vi "log_data_calibration.vi"(0 "Calibration":T1, 3 "error in (no error)":errorcluster, 4 "Elements Remaining":u32, 5 "Data":fxp<+/-,24,4>[](array[numeric])) -> (7 "number of elements out":u32, 10 "error out":errorcluster)   [LabVIEW 2015]
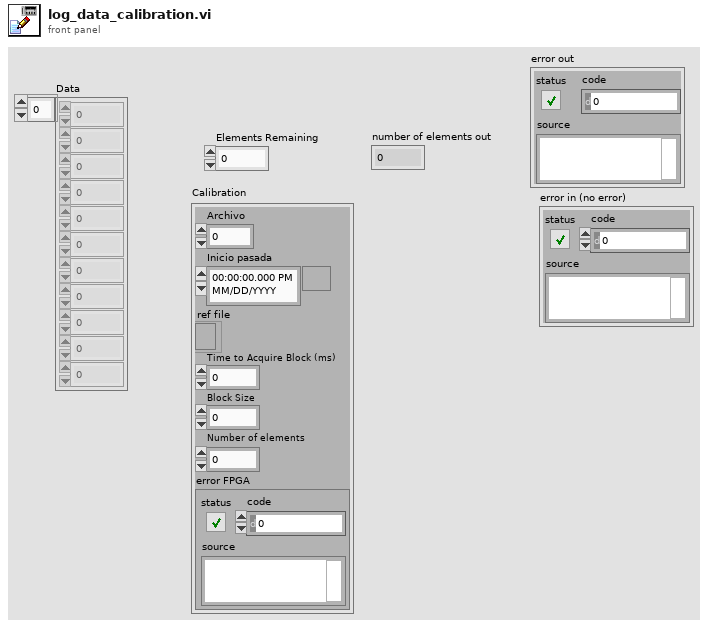
[diagram p1: front panel]
types:
  T1 = cluster{"Archivo":dbl, "Inicio pasada ":timestamp, "ref file":refnum<file>, "Time to Acquire Block (ms)":i32, "Block Size":u32, "Number of elements":u32, "error FPGA":errorcluster}
  T2 = enum16{"big-endian, network order", "native, host order", "little-endian"}
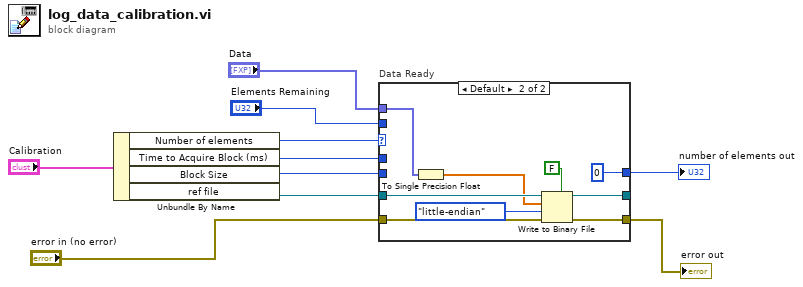
[diagram p0: block diagram]
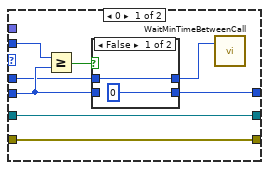
[diagram p2: hidden frame]
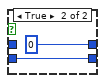
[diagram p3: hidden frame]
diagram:
  n1 = Unbundle By Name("Calibration") -> ("Number of elements"=w6:u32, "Time to Acquire Block (ms)"=w5:i32, "Block Size"=w4:u32, "ref file"=w3:refnum<file>)
  n2 = case "Data Ready" shown="Default" w6 {
    tunnel: w5 -> [w15 _]
    tunnel: [w14 u32 0 ("t")] -> w10
    tunnel: w4 -> [w16 _]
    tunnel: "Elements Remaining" -> [w13 _]
    tunnel: "Data" -> [_ w26]
    tunnel: "error in (no error)" -> [w12 w28]
    tunnel: [w12 w27] -> w2
    tunnel: w3 -> [w11 w25]
    tunnel: [w11 w24] -> _
    frame 0 {
      n3 = Greater Or Equal?(x=w13, y=w16) -> (x >= y?=w17:bool)
      n4 = case shown="False" w17 {
        tunnel: [u32 0 ("Block Size") w21] -> w14
        tunnel: [w20 0 ("t")] -> w18
        tunnel: w15 -> [w20 _]
        tunnel: w16 -> [_ w21]
        frame False {
        }
        frame True {
        }
      }
      n5 = call "WaitMinTimeBetweenCall.vi"("Minimum ms between calls"=w18) -> ()  [unwired: 2 in]
    }
    frame Default {
      n6 = To Single Precision Float(number=w26) -> (single precision float=w23:sgl[])
      n7 = Write to Binary File(file (use dialog)=w25, data=w23, error in=w28, 5:FALSE ("prepend array or string size? (T)"), 9:T2."little-endian" ("byte order (0:big-endian, network order)")) -> (refnum out=w24:refnum<file>, error out=w27:errorcluster)  [unwired: 2 out]
    }
  }
  "number of elements out" <- w10
  "error out" <- w2
